vi "write_dataKyle.vi"(5 "Root Path":path, 6 "File Open In":bool, 7 "RefNum In":refnum<file>, 8 "Data":i16[](array[numeric]), 9 "Bird Name":string, 10 "N Files In":i16) -> (0 "RefNum Out":refnum<file>, 1 "Output File Path":path, 3 "N Files Out":i16, 4 "File Open Out":bool)   [LabVIEW 2010]
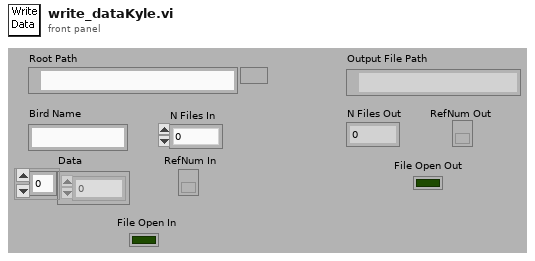
[diagram p1: front panel]
types:
  T1 = enum16{"open", "open or create", "create or replace", "create", "open (read only)"}
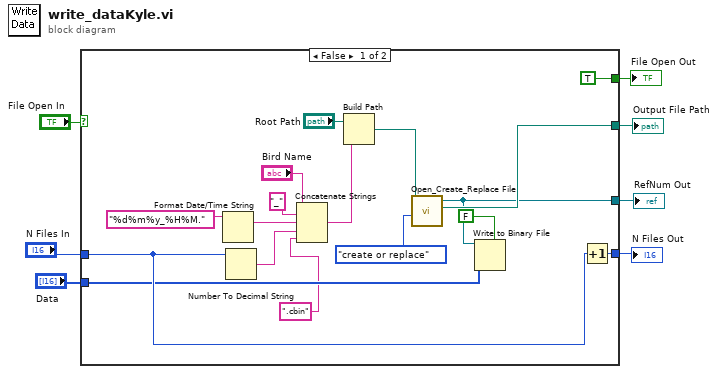
[diagram p0: block diagram]
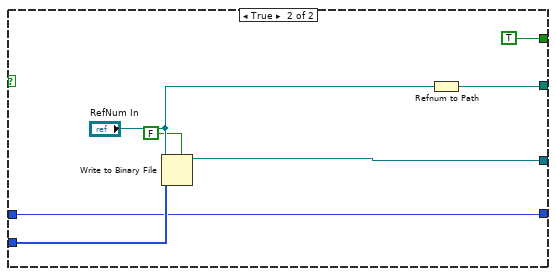
[diagram p2: hidden frame]
diagram:
  n1 = case shown="False" "File Open In" {
    tunnel: "Data" -> [w14 w31]
    tunnel: [w15 w30] -> w1
    tunnel: "N Files In" -> [w20 w29]
    tunnel: [w23 w29] -> w3
    tunnel: [w16 w28] -> w2
    tunnel: [TRUE TRUE] -> w6
    frame False {
      n2 = Format Date/Time String(time format string (%c)="%d%m%y_%H%M.") -> (date/time string=w21:string)  [unwired: 2 in]
      n3 = Number To Decimal String(number=w20) -> (decimal integer string=w19:string)  [unwired: 1 in]
      n4 = Concatenate Strings("Bird Name", "_" ("Substring"), w21, w19, ".cbin" ("Substring")) -> (w18:string)
      n5 = Build Path(base path="Root Path", name or relative path=w18) -> (appended path=w17:path)
      n6 = call <vilib>:"Open_Create_Replace File.vi"("function (open:0)"=T1."create or replace", "file path"=w17) -> ("new file path"=w16:path, "refnum"=w15:refnum<file>)  [unwired: 6 in, 2 out]
      n7 = Write to Binary File(file (use dialog)=w15, data=w14, 5:FALSE ("prepend array or string size? (T)")) -> ()  [unwired: 3 in, 3 out]
      n8 = Increment(x=w20) -> (x+1=w23:i16)
    }
    frame True {
      n9 = Write to Binary File(file (use dialog)="RefNum In", data=w31, 5:FALSE ("prepend array or string size? (T)")) -> (refnum out=w30:refnum<file>)  [unwired: 3 in, 2 out]
      n10 = Refnum to Path(1:"RefNum In") -> (0:w28:path)
    }
  }
  "File Open Out" <- w6
  "N Files Out" <- w3
  "Output File Path" <- w2
  "RefNum Out" <- w1
